vi "Edit_BSA_IP.vi"(3 "Show Panel":bool) -> (1 "Run LDA Diagnostic Out":bool)   [LabVIEW 2010]
uses:
  Globals/Meas_global.vi
  Globals/LDA_meas_global_1.vi
  Globals/LDA_meas_global_2.vi
panel:
  in  "Run LDA Diagnostic":bool
  in  "Bandwidth 0":u16(ring)=11 items=["96.777", "48.389", "24.194", "12.097", "6.049", "3.024", "1.512", "0.756", "0.378", "0.189", "0.095", "0.047"]
  in  "Centre frequency 1":u16(ring)=20 items=["5.378", "5.020", "4.661", "4.303", "3.944", "3.586", "3.227", "2.869", "2.510", "2.151", "1.793", "1.434", "1.076", "0.717", "0.359", "0.000", "-0.359", "-0.717", "-1.076", "-1.434", "-1.793", "-2.151", "-2.510", "-2.869", "-3.227", "-3.586", "-3.944", "-4.303", "-4.661", "-5.020", "-5.378", "-5.737", "-6.096"]
  out "Record Length":dbl[](array[numeric])
  out "Final read?":bool
  in  "OK":bool
  out "C Array":dbl[](array[numeric])
  out "Bandwidth Array Hz":dbl[](array[numeric])
  out "BSA IP Number":string
  out "Using 45 Degree Mirror?":bool
  out "Probe Configuration":string
  out "Focal Length (mm)":dbl
  out "Beam Separation (mm)":dbl
  in  "Bandwidth 1":u16(ring)=11 items=["91.793", "45.896", "22.948", "11.474", "5.737", "2.869", "1.434", "0.717", "0.359", "0.179", "0.090", "0.045"]
  in  "Centre frequency 0":u16(ring)=20 items=["5.671", "5.293", "4.914", "4.536", "4.158", "3.780", "3.402", "3.024", "2.646", "2.268", "1.890", "1.512", "1.134", "0.756", "0.378", "0.000", "-0.378", "-0.756", "-1.134", "-1.512", "-1.890", "-2.268", "-2.646", "-3.024", "-3.402", "-3.780", "-4.158", "-4.536", "-4.914", "-5.293", "-5.671", "-6.049", "-6.427"]
  in  "Setup Array":T1(array[cluster]) {"Bandwidth Hz" format="%.3g"; "Min Record length" items=["16", "32", "64", "128", "256"]; "Optics Conversion Factor" format="%.3g"; "High voltage" min=0 max=2040 step=8; "Signal gain (dB)" min=0 max=30 step=1; "Max Record length" items=["16", "32", "64", "128", "256"]; "Min Velocity" format="%.2g"; "Max Velocity" format="%.2g"; "Wavelength (nm)" format="%.1f"}
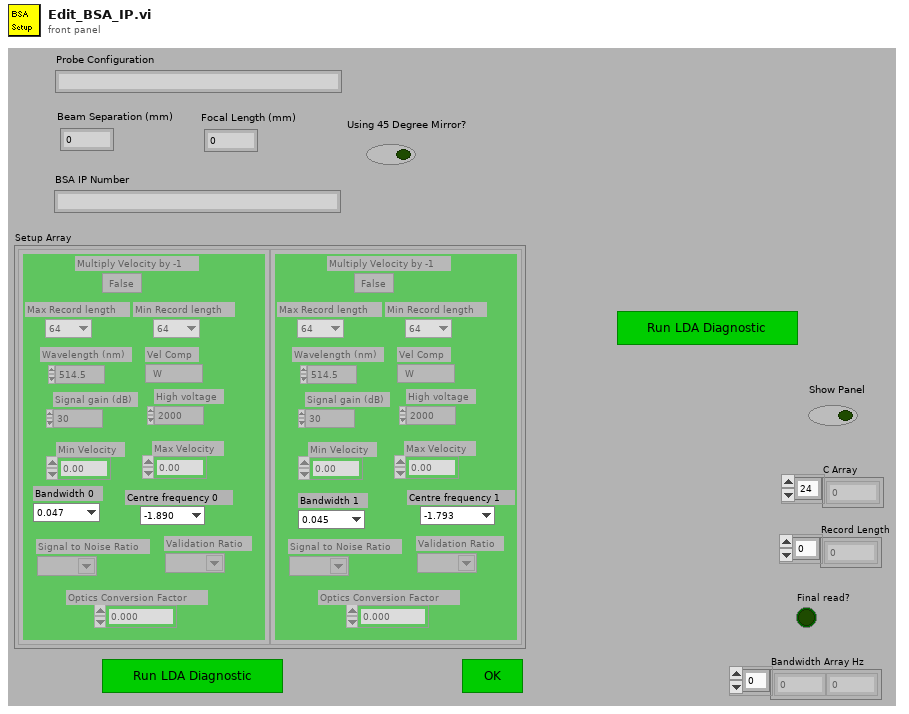
[diagram p1: front panel]
types:
  T1 = cluster{"Wavelength (nm)":dbl, "Vel Comp":string, "Max Velocity":dbl, "Min Velocity":dbl, "COLOUR":u32, "Max Record length":u16, "Signal gain (dB)":i16, "High voltage":i16, "Optics Conversion Factor":dbl, "Min Record length":u16, "Bandwidth Hz":dbl, "Multiply Velocity by -1":bool, "Signal to Noise Ratio":string, "Validation Ratio":string}[]
  T2 = cluster{"Wavelength (nm)":dbl, "Vel Comp":string, "Max Velocity":dbl, "Min Velocity":dbl, "COLOUR":u32, "Max Record length":u16, "Signal gain (dB)":i16, "High voltage":i16, "Optics Conversion Factor":dbl, "Min Record length":u16, "Bandwidth Hz":dbl, "Multiply Velocity by -1":bool, "Signal to Noise Ratio":string, "Validation Ratio":string}
  T3 = typedef "BSA_info_Cluster.ctl" = cluster{"GPIB Address":string, "No of Check Bytes":i32, "Extra Info":string, "COLOUR":u32, "Wavelength (nm)":dbl}
  T4 = typedef "BSA_Type.ctl" = enum16{"57N11", "BSA F60"}
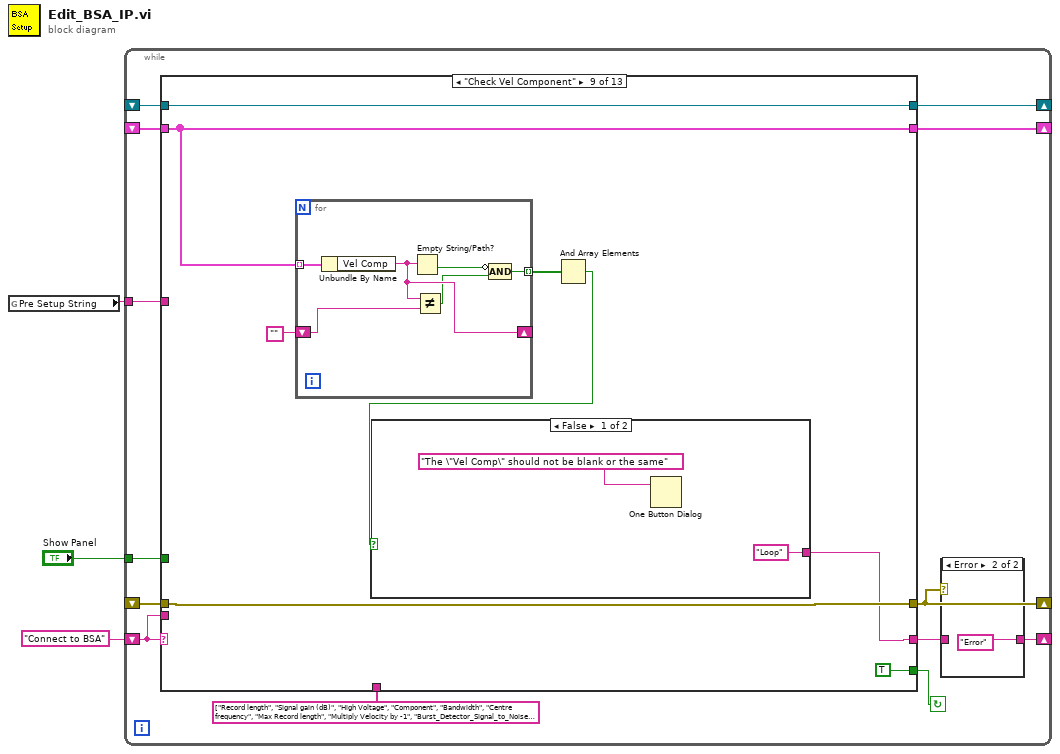
[diagram p0: block diagram]
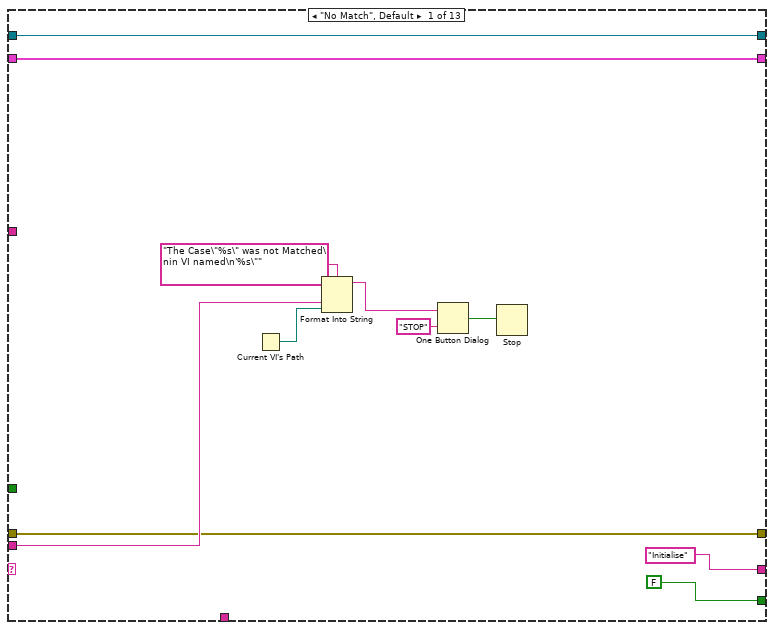
[diagram p3: hidden frame]
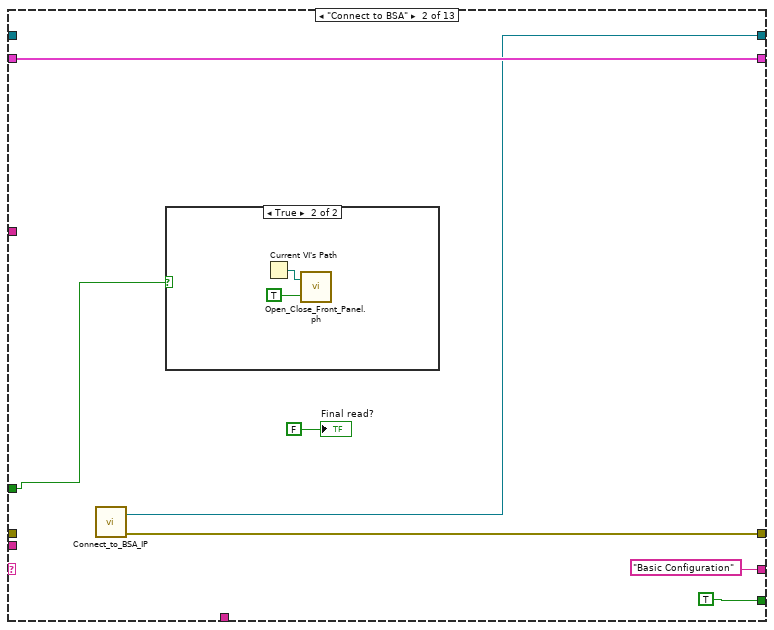
[diagram p4: hidden frame]
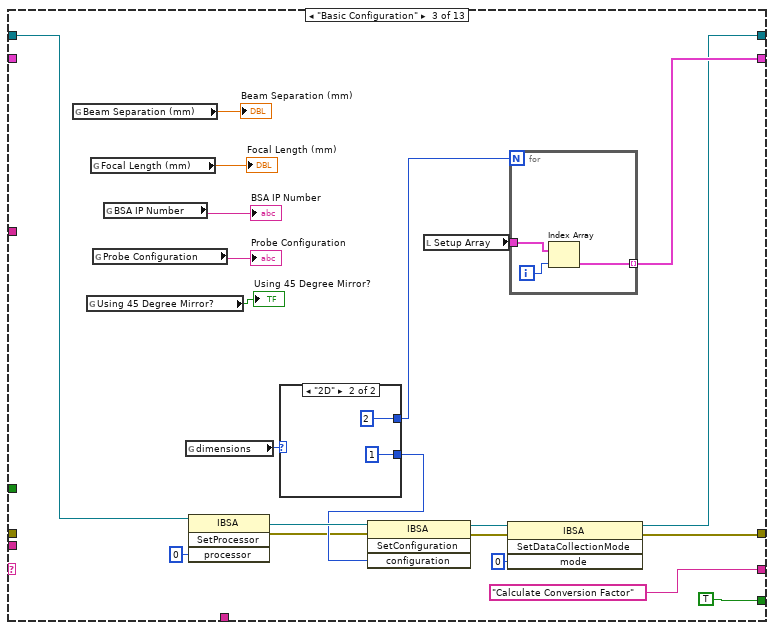
[diagram p6: hidden frame]
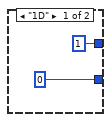
[diagram p7: hidden frame]
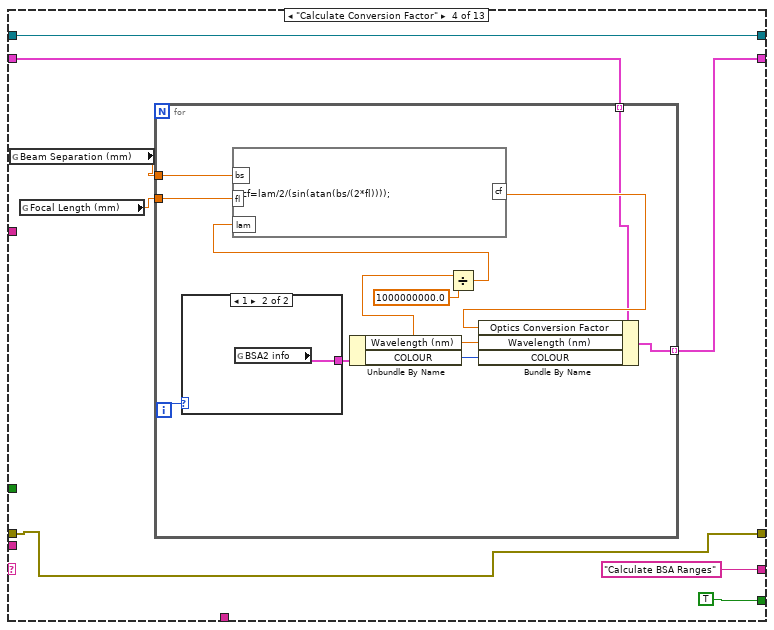
[diagram p8: hidden frame]
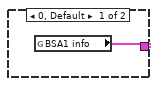
[diagram p9: hidden frame]
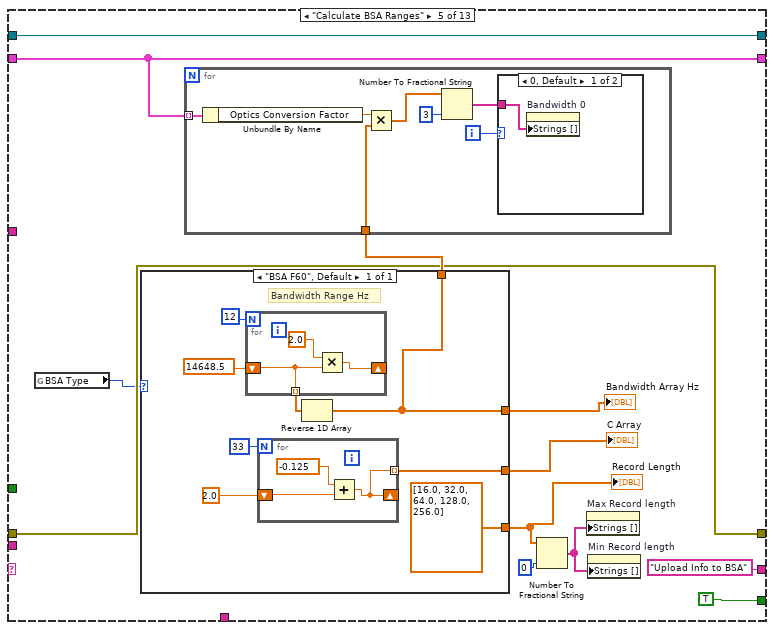
[diagram p10: hidden frame]
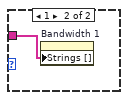
[diagram p11: hidden frame]
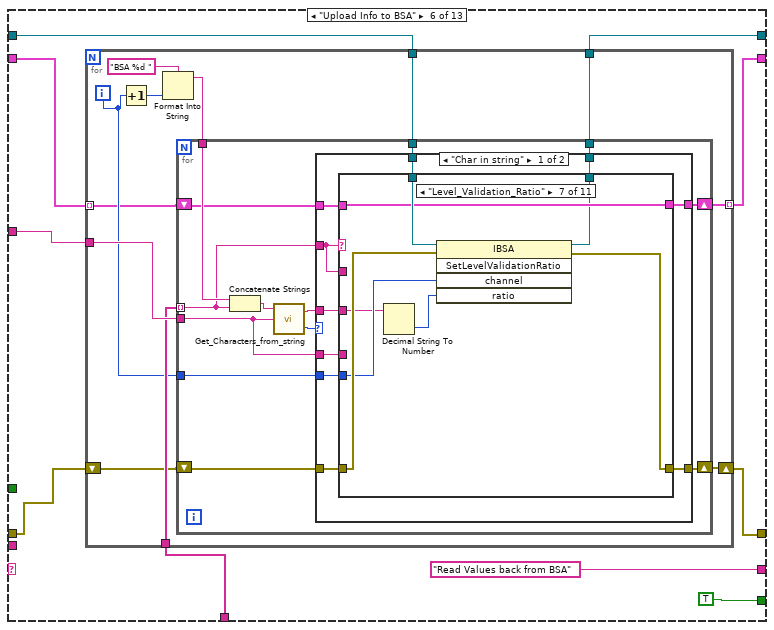
[diagram p12: hidden frame]
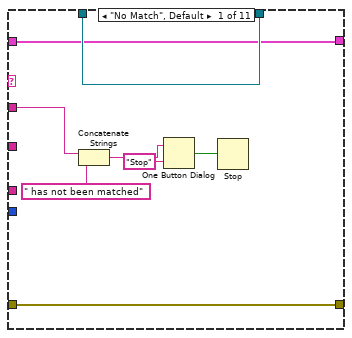
[diagram p13: hidden frame]
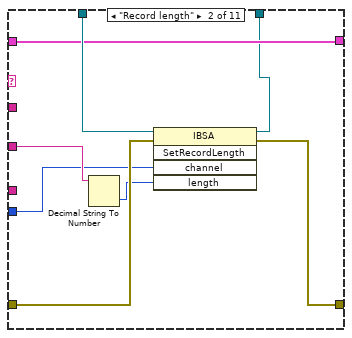
[diagram p14: hidden frame]
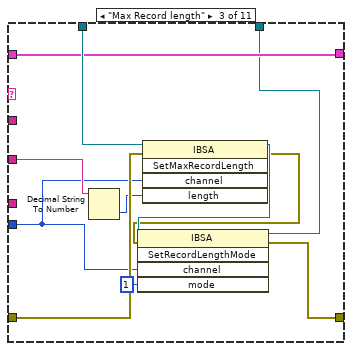
[diagram p15: hidden frame]
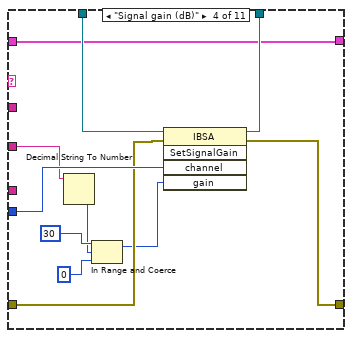
[diagram p16: hidden frame]
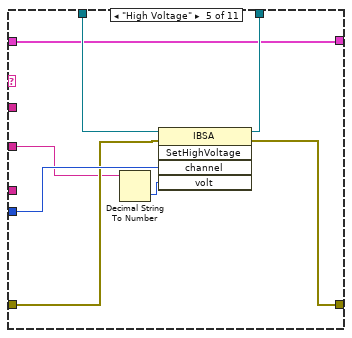
[diagram p17: hidden frame]
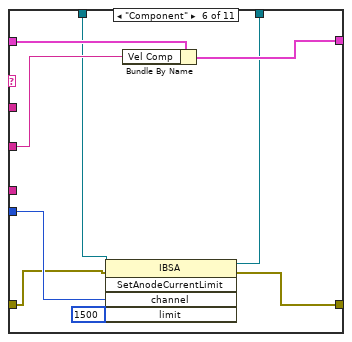
[diagram p18: hidden frame]
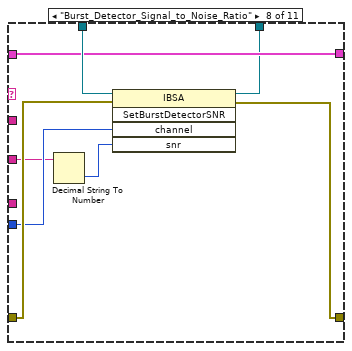
[diagram p19: hidden frame]
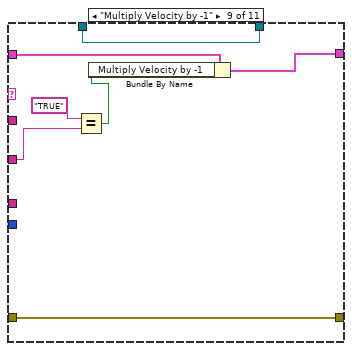
[diagram p20: hidden frame]
diagram:
  n1 = global read "Meas_global.vi" "Pre Setup String"() -> (w2:string)
  n2 = while {
    shift-left: "Connect to BSA" -> [w15]
    shift-right: [w13] -> _
    shift-right: [w11] -> _
    shift-left: _ -> [w9]
    shift-right: [w14] -> _
    shift-left: _ -> [w10]
    tunnel: w2 -> [w8]
    shift-right: [w7] -> _
    shift-left: _ -> [w6]
    tunnel: "Show Panel" -> [w4]
    stop <- w16 continue-if-true
    n3 = case shown="\"Check Vel Component\"" w15 {
      tunnel: [FALSE TRUE TRUE TRUE TRUE TRUE TRUE TRUE TRUE ("Show Panel") TRUE FALSE w609 FALSE] -> w16
      tunnel: ["Initialise" "Basic Configuration" "Calculate Conversion Factor" "Calculate BSA Ranges" "Upload Info to BSA" "Read Values back from BSA" w269 w406 w471 "Read Values back from BSA" "Second Case" "Close Panel" "End" ("f")] -> w12
      tunnel: w15 -> [w24 _ _ _ _ _ _ _ _ _ _ _ _]
      tunnel: [w20 w32 w40 w69 w95 w127 w276 w411 w473 w491 w604 w611 w672] -> w14
      tunnel: [w21 w33 w41 w70 w98 w129 w278 w416 w477 w493 w605 w613 w673] -> w11
      tunnel: w10 -> [w20 _ _ w69 w95 w128 w277 w411 w473 w492 w604 w611 w672]
      tunnel: w9 -> [w21 _ w53 w70 w98 w130 w279 w416 w477 w494 w605 w613 w673]
      tunnel: w8 -> [_ _ _ _ _ w131 w280 _ _ w495 _ _ _]
      tunnel: [w19 w34 w45 w71 w97 w125 w273 w412 w470 w489 w603 w612 w668] -> w7
      tunnel: w6 -> [w19 w34 _ w68 w97 w126 w275 _ w470 w490 w603 w612 w668]
      tunnel: string[] ["Record length", "Signal gain (dB)", "High Voltage", "Component", "Bandwidth", "Centre frequency", "Max Record length", "Multiply Velocity by -1", "Burst_Detector_Signal_to_Noise_Ratio", "Level_Validation_Ratio"] -> [_ _ _ _ _ w124 w274 _ _ w488 _ _ _]
      tunnel: w4 -> [_ w30 _ _ _ _ _ w403 _ _ _ w609 _]
      frame "No Match", Default {
        n4 = Current VI's Path() -> (path=w23:path)
        n5 = Format Into String(format string="The Case\"%s\" was not Matched\nin VI named\n'%s\"" ("Format String"), w24, w23) -> (resulting string=w27:string)  [unwired: 2 in, 1 out]
        n6 = One Button Dialog(message=w27, button name ("OK")="STOP") -> (true=w25:bool)
        n7 = Stop(stop? (T)=w25) -> ()
      }
      frame "Connect to BSA" {
        n8 = call "Connect_to_BSA_IP.vi"() -> ("error out"=w32:errorcluster, "BSA"=w33:refnum<k7>)  [unwired: 2 out]
        n9 = case shown="True" w30 {
          frame False {
          }
          frame True {
            n10 = Current VI's Path() -> (path=w37:path)
            n11 = call "Open_Close_Front_Panel.ph.vi"("Front Panel Window:Open"=TRUE, "VI path"=w37) -> ()  [unwired: 2 out]
          }
        }
        "Final read?" <- FALSE ("Boolean")
      }
      frame "Basic Configuration" {
        n12 = global read "LDA_meas_global_1.vi" "Beam Separation (mm)"() -> (→"Beam Separation (mm)":dbl)
        n13 = global read "LDA_meas_global_1.vi" "Using 45 Degree Mirror?"() -> (→"Using 45 Degree Mirror?":bool)
        n14 = global read "LDA_meas_global_1.vi" "Focal Length (mm)"() -> (→"Focal Length (mm)":dbl)
        n15 = global read "LDA_meas_global_1.vi" "Probe Configuration"() -> (→"Probe Configuration":string)
        n16 = global read "LDA_meas_global_1.vi" "BSA IP Number"() -> (→"BSA IP Number":string)
        n17 = global read "Meas_global.vi" "dimensions"() -> (w56:enum16{"1D", "2D"})
        n18 = invoke class="IBSA" method="SetProcessor"(reference=w53, "processor"=0) -> (reference out=w57:refnum<k7>, error out=w54:errorcluster)  [unwired: 2 in, 2 out]
        n19 = case shown="\"2D\"" w56 {
          tunnel: [0 ("config") 1 ("config")] -> w55
          tunnel: [1 2] -> w46
          frame "1D" {
          }
          frame "2D" {
          }
        }
        n20 = invoke class="IBSA" method="SetConfiguration"(reference=w57, error in=w54, "configuration"=w55) -> (reference out=w43:refnum<k7>, error out=w42:errorcluster)  [unwired: 1 in, 2 out]
        n21 = local read "Setup Array"() -> (w47:T1)
        n22 = invoke class="IBSA" method="SetDataCollectionMode"(reference=w43, error in=w42, "mode"=0) -> (reference out=w41:refnum<k7>, error out=w40:errorcluster)  [unwired: 1 in, 2 out]
        n23 = for {
          N: w46 -> [_]
          tunnel: w47 -> [w61]
          tunnel: [w60] -> w45 mode=indexing
          i -> [w62]
          n24 = Index Array(array=w61, index=w62) -> (element=w60:T2)
        }
      }
      frame "Calculate Conversion Factor" {
        n25 = global read "LDA_meas_global_1.vi" "Beam Separation (mm)"() -> (w72:dbl)
        n26 = global read "LDA_meas_global_1.vi" "Focal Length (mm)"() -> (w73:dbl)
        n27 = for {
          tunnel: w72 -> [w85]
          tunnel: w73 -> [w84]
          tunnel: [w76] -> w71 mode=indexing
          tunnel: w68 -> [w75] mode=indexing
          i -> [w82]
          n28 = case shown="1" w82 {
            tunnel: [w86 w87] -> w83
            frame 0, Default {
              n29 = global read "LDA_meas_global_1.vi" "BSA1 info"() -> (w86:T3)
            }
            frame 1 {
              n30 = global read "LDA_meas_global_2.vi" "BSA2 info"() -> (w87:T3)
            }
          }
          n31 = Unbundle By Name(w83) -> ("Wavelength (nm)"=w79:dbl, "COLOUR"=w81:u32)
          n32 = Divide(x=w79, y=1000000000.0) -> (x/y=w77:dbl)
          n33 = formula code="cf=lam/2/(sin(atan(bs/(2*fl))));"("bs"=w85, "fl"=w84, "lam"=w77) -> ("cf"=w80:dbl)
          n34 = Bundle By Name(cluster=w75, "Optics Conversion Factor"=w80, "Wavelength (nm)"=w79, "COLOUR"=w81) -> (w76:T2)
        }
      }
      frame "Calculate BSA Ranges" {
        n35 = global read "LDA_meas_global_1.vi" "BSA Type"() -> (w89:T4)
        n36 = case shown="\"BSA F60\", Default" w89 {
          tunnel: [w110] -> w96
          tunnel: [w111] -> w93
          tunnel: [w110] -> w92
          tunnel: [dbl[] [16.0, 32.0, 64.0, 128.0, 256.0] ("Max Record Length")] -> w90
          frame "BSA F60", Default {
            # "Bandwidth Range Hz"
            n37 = for {
              N: 12 -> [_]
              shift-right: [w122] -> _
              shift-left: 14648.5 -> [w120]
              tunnel: [w120] -> w114 mode=indexing
              n38 = Multiply(x=2.0, y=w120) -> (x*y=w122:dbl)
            }
            n39 = for {
              N: 33 -> [_]
              shift-right: [w117] -> _
              shift-left: 2.0 -> [w119]
              tunnel: [w117] -> w111 mode=indexing
              n40 = Add(x=-0.125, y=w119) -> (x+y=w117:dbl)
            }
            n41 = Reverse 1D Array(array=w114) -> (reversed array=w110:dbl[])
          }
        }
        "C Array" <- w93
        "Bandwidth Array Hz" <- w92
        "Record Length" <- w90
        n42 = for {
          tunnel: w97 -> [w106] mode=indexing
          tunnel: w96 -> [w104]
          i -> [w105]
          n43 = Unbundle By Name(w106) -> ("Optics Conversion Factor"=w100:dbl)
          n44 = Multiply(x=w100, y=w104) -> (x*y=w103:dbl[])
          n45 = Number To Fractional String(number=w103, precision (6)=i16 3) -> (F-format string=w101:string[])  [unwired: 2 out]
          n46 = case shown="0, Default" w105 {
            tunnel: w101 -> [w107 w108]
            frame 0, Default {
              n47 = property on="Bandwidth 0" class="Ring (strict)"("Strings []"=w107) -> ()  [unwired: 2 in, 2 out]
            }
            frame 1 {
              n48 = property on="Bandwidth 1" class="Ring (strict)"("Strings []"=w108) -> ()  [unwired: 2 in, 2 out]
            }
          }
        }
        n49 = Number To Fractional String(number=w90, precision (6)=i16 0) -> (F-format string=w88:string[])  [unwired: 2 out]
        n50 = property on="Max Record length" class="Ring (strict)"("Strings []"=w88) -> ()  [unwired: 2 in, 2 out]
        n51 = property on="Min Record length" class="Ring (strict)"("Strings []"=w88) -> ()  [unwired: 2 in, 2 out]
      }
      frame "Upload Info to BSA" {
        n52 = for {
          tunnel: w131 -> [w144]
          tunnel: w130 -> [w143]
          tunnel: [w142] -> w129
          shift-right: [w139] -> w127
          shift-left: w128 -> [w140]
          tunnel: w124 -> [w141]
          tunnel: w126 -> [w134] mode=indexing
          tunnel: [w133] -> w125 mode=indexing
          i -> [w138]
          n53 = Increment(x=w138) -> (x+1=w137:i32)
          n54 = Format Into String(format string="BSA %d ", w137) -> (resulting string=w135:string)  [unwired: 2 in, 1 out]
          n55 = for {
            tunnel: w135 -> [w157]
            tunnel: w138 -> [w156]
            tunnel: w144 -> [w149]
            tunnel: w143 -> [w155]
            tunnel: [w154] -> w142
            tunnel: w141 -> [w153] mode=indexing
            shift-right: [w151] -> w139
            shift-left: w140 -> [w152]
            shift-right: [w145] -> w133
            shift-left: w134 -> [w146]
            n56 = Concatenate Strings(w157, w153) -> (w150:string)
            n57 = call "Get_Characters_from_string.vi"("Input string"=w149, "Variable name"=w150) -> ("Status"=w148:enum16{"Char in string", "Char not in string"}, "Value"=w147:string)  [unwired: 1 in]
            n58 = case shown="\"Char in string\"" w148 {
              tunnel: w156 -> [w167 _]
              tunnel: w147 -> [w166 _]
              tunnel: w153 -> [w161 _]
              tunnel: w155 -> [w165 w268]
              tunnel: [w164 w268] -> w154
              tunnel: [w163 w267] -> w151
              tunnel: w152 -> [w162 w267]
              tunnel: w146 -> [w160 w266]
              tunnel: w149 -> [w159 _]
              tunnel: [w158 w266] -> w145
              frame "Char in string" {
                n59 = case shown="\"Level_Validation_Ratio\"" w161 {
                  tunnel: w167 -> [_ w178 w188 w205 w213 w219 w228 w236 _ w255 w265]
                  tunnel: w166 -> [_ w181 w192 w200 w207 w221 w226 w234 w243 w250 w260]
                  tunnel: w165 -> [w175 w183 w194 w204 w212 w215 w230 w238 w239 w254 w264]
                  tunnel: [w175 w177 w184 w203 w211 w216 w223 w231 w239 w253 w263] -> w164
                  tunnel: [w174 w176 w185 w202 w210 w217 w224 w232 w240 w252 w262] -> w163
                  tunnel: w162 -> [w174 w182 w193 w201 w209 w214 w229 w237 w240 w251 w261]
                  tunnel: w161 -> [w173 _ _ _ _ _ _ _ _ _ _]
                  tunnel: w160 -> [w168 w180 w191 w199 w206 w222 w227 w235 w245 w248 w258]
                  tunnel: w159 -> [_ _ _ _ _ _ _ _ _ _ _]
                  tunnel: [w168 w180 w191 w199 w206 w220 w227 w235 w244 w248 w258] -> w158
                  frame "No Match", Default {
                    n60 = Concatenate Strings(w173, " has not been matched" ("string")) -> (w171:string)
                    n61 = One Button Dialog(message=w171, button name ("OK")="Stop") -> (true=w169:bool)
                    n62 = Stop(stop? (T)=w169) -> ()
                  }
                  frame "Record length" {
                    n63 = Decimal String To Number(string=w181) -> (number=w179:i32)  [unwired: 3 out]
                    n64 = invoke class="IBSA" method="SetRecordLength"(reference=w183, error in=w182, "channel"=w178, "length"=w179) -> (reference out=w177:refnum<k7>, error out=w176:errorcluster)  [unwired: 1 in, 3 out]
                  }
                  frame "Max Record length" {
                    n65 = Decimal String To Number(string=w192) -> (number=w190:i32)  [unwired: 3 out]
                    n66 = invoke class="IBSA" method="SetMaxRecordLength"(reference=w194, error in=w193, "channel"=w188, "length"=w190) -> (reference out=w187:refnum<k7>, error out=w186:errorcluster)  [unwired: 1 in, 3 out]
                    n67 = invoke class="IBSA" method="SetRecordLengthMode"(reference=w187, error in=w186, "channel"=w188, "mode"=1) -> (reference out=w184:refnum<k7>, error out=w185:errorcluster)  [unwired: 1 in, 3 out]
                  }
                  frame "Signal gain (dB)" {
                    n68 = Decimal String To Number(string=w200) -> (number=w195:i32)  [unwired: 3 out]
                    n69 = In Range and Coerce(upper limit=30, x=w195, lower limit=0) -> (coerced(x)=w196:i32)  [unwired: 1 out]
                    n70 = invoke class="IBSA" method="SetSignalGain"(reference=w204, error in=w201, "channel"=w205, "gain"=w196) -> (reference out=w203:refnum<k7>, error out=w202:errorcluster)  [unwired: 1 in, 3 out]
                  }
                  frame "High Voltage" {
                    n71 = Decimal String To Number(string=w207) -> (number=w208:i32)  [unwired: 3 out]
                    n72 = invoke class="IBSA" method="SetHighVoltage"(reference=w212, error in=w209, "channel"=w213, "volt"=w208) -> (reference out=w211:refnum<k7>, error out=w210:errorcluster)  [unwired: 1 in, 3 out]
                  }
                  frame "Component" {
                    n73 = invoke class="IBSA" method="SetAnodeCurrentLimit"(reference=w215, error in=w214, "channel"=w219, "limit"=1500) -> (reference out=w216:refnum<k7>, error out=w217:errorcluster)  [unwired: 1 in, 3 out]
                    n74 = Bundle By Name(cluster=w222, "Vel Comp"=w221) -> (w220:T2)
                  }
                  frame "Level_Validation_Ratio" {
                    n75 = Decimal String To Number(string=w226) -> (number=w225:i32)  [unwired: 3 out]
                    n76 = invoke class="IBSA" method="SetLevelValidationRatio"(reference=w230, error in=w229, "channel"=w228, "ratio"=w225) -> (reference out=w223:refnum<k7>, error out=w224:errorcluster)  [unwired: 1 in, 3 out]
                  }
                  frame "Burst_Detector_Signal_to_Noise_Ratio" {
                    n77 = Decimal String To Number(string=w234) -> (number=w233:i32)  [unwired: 3 out]
                    n78 = invoke class="IBSA" method="SetBurstDetectorSNR"(reference=w238, error in=w237, "channel"=w236, "snr"=w233) -> (reference out=w231:refnum<k7>, error out=w232:errorcluster)  [unwired: 1 in, 3 out]
                  }
                  frame "Multiply Velocity by -1" {
                    n79 = Equal?(x="TRUE", y=w243) -> (x = y?=w241:bool)
                    n80 = Bundle By Name(cluster=w245, "Multiply Velocity by -1"=w241) -> (w244:T2)
                  }
                  frame "Bandwidth" {
                    n81 = Fract/Exp String To Number(string=w250) -> (number=w249:dbl)  [unwired: 4 out]
                    n82 = Unbundle By Name(w248) -> ("Optics Conversion Factor"=w247:dbl)
                    n83 = Divide(x=w249, y=w247) -> (x/y=w246:dbl)
                    n84 = invoke class="IBSA" method="SetBandwidth"(reference=w254, error in=w251, "channel"=w255, "bandwidth"=w246) -> (reference out=w253:refnum<k7>, error out=w252:errorcluster)  [unwired: 1 in, 3 out]
                  }
                  frame "Centre frequency" {
                    n85 = Fract/Exp String To Number(string=w260) -> (number=w259:dbl)  [unwired: 4 out]
                    n86 = Unbundle By Name(w258) -> ("Optics Conversion Factor"=w257:dbl)
                    n87 = Divide(x=w259, y=w257) -> (x/y=w256:dbl)
                    n88 = invoke class="IBSA" method="SetCenterFreq"(reference=w264, error in=w261, "channel"=w265, "freq"=w256) -> (reference out=w263:refnum<k7>, error out=w262:errorcluster)  [unwired: 1 in, 3 out]
                  }
                }
              }
              frame "Char not in string" {
              }
            }
          }
        }
      }
      frame "Read Values back from BSA" {
        n89 = for {
          tunnel: w280 -> [w290]
          tunnel: w279 -> [w289]
          tunnel: [w288] -> w278
          shift-right: [w285] -> w276
          shift-left: w277 -> [w286]
          tunnel: w274 -> [w287]
          tunnel: w275 -> [w284] mode=indexing
          tunnel: [w283] -> w273 mode=indexing
          i -> [w282]
          n90 = for {
            tunnel: w282 -> [w299]
            tunnel: w290 -> [w293]
            tunnel: w289 -> [w298]
            tunnel: [w297] -> w288
            tunnel: w287 -> [w296] mode=indexing
            shift-right: [w294] -> w285
            shift-left: w286 -> [w295]
            shift-right: [w291] -> w283
            shift-left: w284 -> [w292]
            n91 = case shown="\"Level_Validation_Ratio\"" w296 {
              tunnel: w299 -> [_ w319 w331 w339 w348 w357 w365 _ _ w379 w394]
              tunnel: w298 -> [w307 w318 w330 w338 w347 w356 w364 w367 w370 w383 w398]
              tunnel: [w307 w317 w329 w337 w346 w355 w363 w367 w370 w382 w397] -> w297
              tunnel: [w306 w316 w328 w336 w345 w354 w362 w368 w371 w381 w396] -> w294
              tunnel: w295 -> [w306 w315 w327 w335 w344 w353 w361 w368 w371 w380 w395]
              tunnel: w296 -> [w305 _ _ _ _ _ _ _ _ _ _]
              tunnel: w292 -> [w300 w314 w326 w333 w343 w352 w360 w366 w369 w374 w390]
              tunnel: w293 -> [_ _ _ _ _ _ _ _ _ _ _]
              tunnel: [w300 w313 w325 w332 w342 w351 w359 w366 w369 w372 w390] -> w291
              frame "No Match", Default {
                n92 = Concatenate Strings(w305, " has not been matched" ("string")) -> (w303:string)
                n93 = One Button Dialog(message=w303, button name ("OK")="Stop") -> (true=w301:bool)
                n94 = Stop(stop? (T)=w301) -> ()
              }
              frame "Record length" {
                n95 = local read "Record Length"() -> (w310:dbl[])
                n96 = invoke class="IBSA" method="GetRecordLength"(reference=w318, error in=w315, "channel"=w319) -> (reference out=w317:refnum<k7>, error out=w316:errorcluster, "GetRecordLength"=w309:i32)  [unwired: 1 in, 1 out]
                n97 = Subtract(x=w310, y=w309) -> (x-y=w312:dbl[])
                n98 = Absolute Value(x=w312) -> (abs(x)=w311:dbl[])
                n99 = Array Max & Min(array=w311) -> (min index (indices)=w308:i32)  [unwired: 3 out]
                n100 = Bundle By Name(cluster=w314, "Min Record length"=w308) -> (w313:T2)
              }
              frame "Max Record length" {
                n101 = local read "Record Length"() -> (w322:dbl[])
                n102 = invoke class="IBSA" method="GetMaxRecordLength"(reference=w330, error in=w327, "channel"=w331) -> (reference out=w329:refnum<k7>, error out=w328:errorcluster, "GetMaxRecordLength"=w321:i32)  [unwired: 1 in, 1 out]
                n103 = Subtract(x=w322, y=w321) -> (x-y=w324:dbl[])
                n104 = Absolute Value(x=w324) -> (abs(x)=w323:dbl[])
                n105 = Array Max & Min(array=w323) -> (min index (indices)=w320:i32)  [unwired: 3 out]
                n106 = Bundle By Name(cluster=w326, "Max Record length"=w320) -> (w325:T2)
              }
              frame "Signal gain (dB)" {
                n107 = invoke class="IBSA" method="GetSignalGain"(reference=w338, error in=w335, "channel"=w339) -> (reference out=w337:refnum<k7>, error out=w336:errorcluster, "GetSignalGain"=w334:i32)  [unwired: 1 in, 1 out]
                n108 = Bundle By Name(cluster=w333, "Signal gain (dB)"=w334) -> (w332:T2)
              }
              frame "Burst_Detector_Signal_to_Noise_Ratio" {
                n109 = invoke class="IBSA" method="GetBurstDetectorSNR"(reference=w347, error in=w344, "channel"=w348) -> (reference out=w346:refnum<k7>, error out=w345:errorcluster, "GetBurstDetectorSNR"=w340:i32)  [unwired: 1 in, 1 out]
                n110 = Number To Decimal String(number=w340) -> (decimal integer string=w341:string)  [unwired: 1 out]
                n111 = Bundle By Name(cluster=w343, "Signal to Noise Ratio"=w341) -> (w342:T2)
              }
              frame "Level_Validation_Ratio" {
                n112 = invoke class="IBSA" method="GetLevelValidationRatio"(reference=w356, error in=w353, "channel"=w357) -> (reference out=w355:refnum<k7>, error out=w354:errorcluster, "GetLevelValidationRatio"=w349:i32)  [unwired: 1 in, 1 out]
                n113 = Number To Decimal String(number=w349) -> (decimal integer string=w350:string)  [unwired: 1 out]
                n114 = Bundle By Name(cluster=w352, "Validation Ratio"=w350) -> (w351:T2)
              }
              frame "High Voltage" {
                n115 = invoke class="IBSA" method="GetHighVoltage"(reference=w364, error in=w361, "channel"=w365) -> (reference out=w363:refnum<k7>, error out=w362:errorcluster, "GetHighVoltage"=w358:i32)  [unwired: 1 in, 1 out]
                n116 = Bundle By Name(cluster=w360, "High voltage"=w358) -> (w359:T2)
              }
              frame "Component" {
              }
              frame "Multiply Velocity by -1" {
              }
              frame "Bandwidth" {
                n117 = local read "Bandwidth Array Hz"() -> (w376:dbl[])
                n118 = invoke class="IBSA" method="GetBandwidth"(reference=w383, error in=w380, "channel"=w379) -> (reference out=w382:refnum<k7>, error out=w381:errorcluster, "GetBandwidth"=w373:sgl)  [unwired: 1 in, 1 out]
                n119 = Bundle By Name(cluster=w374, "Bandwidth Hz"=w373) -> (w372:T2)
                n120 = Subtract(x=w376, y=w373) -> (x-y=w378:dbl[])
                n121 = Absolute Value(x=w378) -> (abs(x)=w377:dbl[])
                n122 = Array Max & Min(array=w377) -> (min index (indices)=w375:i32)  [unwired: 3 out]
                n123 = case shown="1" w379 {
                  tunnel: w375 -> [w384 w385]
                  frame 0, Default {
                    n124 = local write "Bandwidth 0"(w384) -> ()
                  }
                  frame 1 {
                    n125 = local write "Bandwidth 1"(w385) -> ()
                  }
                }
              }
              frame "Centre frequency" {
                n126 = local read "C Array"() -> (w389:dbl[])
                n127 = Unbundle By Name(w390) -> ("Bandwidth Hz"=w387:dbl)
                n128 = invoke class="IBSA" method="GetCenterFreq"(reference=w398, error in=w395, "channel"=w394) -> (reference out=w397:refnum<k7>, error out=w396:errorcluster, "GetCenterFreq"=w388:sgl)  [unwired: 1 in, 1 out]
                n129 = Divide(x=w388, y=w387) -> (x/y=w386:dbl)
                n130 = Subtract(x=w389, y=w386) -> (x-y=w393:dbl[])
                n131 = Absolute Value(x=w393) -> (abs(x)=w392:dbl[])
                n132 = Array Max & Min(array=w392) -> (min index (indices)=w391:i32)  [unwired: 3 out]
                n133 = case shown="1" w394 {
                  tunnel: w391 -> [w399 w400]
                  frame 0, Default {
                    n134 = local write "Centre frequency 0"(w399) -> ()
                  }
                  frame 1 {
                    n135 = local write "Centre frequency 1"(w400) -> ()
                  }
                }
              }
            }
          }
        }
        n136 = local read "Final read?"() -> (w272:bool)
        n137 = local write "Setup Array"(w273) -> ()
        n138 = Select(t="Update Globals", s=w272, f="Loop") -> (s? t:f=w269:string)
      }
      frame "Loop" {
        n139 = local read "Bandwidth Array Hz"() -> (w415:dbl[])
        n140 = local read "C Array"() -> (w414:dbl[])
        n141 = Wait Until Next ms Multiple(millisecond multiple=u32 300) -> ()  [unwired: 1 out]
        n142 = for {
          tunnel: w415 -> [w445]
          tunnel: w414 -> [w427]
          tunnel: [w442] -> w412 mode=indexing
          tunnel: "Setup Array" -> [w432] mode=indexing
          i -> [w441]
          n143 = Unbundle By Name(w432) -> ("Optics Conversion Factor"=w440:dbl, "Max Record length"=w433:u16, "Min Record length"=w435:u16, "Multiply Velocity by -1"=w426:bool)
          n144 = case shown="1" w441 {
            tunnel: ["Bandwidth 0" "Bandwidth 1"] -> w446
            tunnel: ["Centre frequency 0" "Centre frequency 1"] -> w444
            frame 0, Default {
            }
            frame 1 {
            }
          }
          n145 = Greater Or Equal?(x=w433, y=w435) -> (x >= y?=w434:bool)
          n146 = case shown="False" w434 {
            tunnel: w432 -> [w458 w459]
            tunnel: w433 -> [w457 _]
            tunnel: [w456 w459] -> w431
            frame False {
              n147 = Bundle By Name(cluster=w458, "Min Record length"=w457) -> (w456:T2)
            }
            frame True {
            }
          }
          n148 = Index Array(array=w445, index=w446) -> (element=w439:dbl)
          n149 = Multiply(x=w440, y=w439) -> (x*y=w437:dbl)
          n150 = Multiply(x=w427, y=w437) -> (x*y=w423:dbl[])
          n151 = Index Array(array=w423, index=w444) -> (element=w428:dbl)
          n152 = Divide(x=w437, y=2.0) -> (x/y=w429:dbl)
          n153 = Negate(x=w429) -> (-x=w430:dbl)
          n154 = Add(x=w430, y=w428) -> (x+y=w424:dbl)
          n155 = Add(x=w429, y=w428) -> (x+y=w425:dbl)
          n156 = case shown="False" w426 {
            tunnel: [w447 w453] -> w418
            tunnel: w425 -> [w447 w455]
            tunnel: [w449 w452] -> w419
            tunnel: w424 -> [w449 w454]
            tunnel: w423 -> [w448 w451]
            tunnel: [w448 w450] -> w422
            frame False {
            }
            frame True {
              n157 = Negate(x=w454) -> (-x=w452:dbl)
              n158 = Negate(x=w455) -> (-x=w453:dbl)
              n159 = Negate(x=w451) -> (-x=w450:dbl[])
            }
          }
          n160 = Max & Min(x=w419, y=w418) -> (max(x,y)=w420:dbl, min(x,y)=w421:dbl)
          n161 = Bundle By Name(cluster=w431, "Max Velocity"=w420, "Min Velocity"=w421) -> (w442:T2)
          n162 = Number To Fractional String(number=w422, precision (6)=i16 3) -> (F-format string=w436:string[])  [unwired: 2 out]
          n163 = case shown="1" w441 {
            tunnel: w437 -> [w462 w465]
            tunnel: w428 -> [w461 w464]
            tunnel: w436 -> [w460 w463]
            frame 0, Default {
              n164 = global write "LDA_meas_global_1.vi" "Centre Freq BSA1"(w461) -> ()
              n165 = global write "LDA_meas_global_1.vi" "Bandwidth BSA1"(w462) -> ()
              n166 = property on="Centre frequency 0" class="Ring (strict)"("Strings []"=w460) -> ()  [unwired: 2 in, 2 out]
            }
            frame 1 {
              n167 = global write "LDA_meas_global_2.vi" "Centre Freq BSA2"(w464) -> ()
              n168 = global write "LDA_meas_global_2.vi" "Bandwidth BSA2"(w465) -> ()
              n169 = property on="Centre frequency 1" class="Ring (strict)"("Strings []"=w463) -> ()  [unwired: 2 in, 2 out]
            }
          }
        }
        n170 = Not Equal?(x=w412, y="Setup Array") -> (x != y?=w413:bool)
        n171 = case shown="True" w413 {
          tunnel: w412 -> [_ w417]
          frame False {
          }
          frame True {
            n172 = local write "Setup Array"(w417) -> ()
          }
        }
        n173 = Compound Arithmetic op=AND(invert "Run LDA Diagnostic", invert "OK", w403) -> (w407:bool)
        n174 = Select(t="Loop", s=w407, f="Check Vel Component") -> (s? t:f=w406:string)
        "Run LDA Diagnostic Out" <- "Run LDA Diagnostic"
      }
      frame "Check Vel Component" {
        n175 = for {
          tunnel: w470 -> [w486] mode=indexing
          shift-right: [w484] -> _
          shift-left: "" -> [w485]
          tunnel: [w481] -> w475 mode=indexing
          n176 = Unbundle By Name(w486) -> ("Vel Comp"=w484:string)
          n177 = Empty String/Path?(string/path=w484) -> (empty?=w483:bool)
          n178 = Not Equal?(x=w484, y=w485) -> (x != y?=w482:bool)
          n179 = Compound Arithmetic op=AND(invert w483, w482) -> (w481:bool)
        }
        n180 = And Array Elements(Boolean array=w475) -> (logical AND=w474:bool)
        n181 = case shown="False" w474 {
          tunnel: ["Loop" "Write Setup to BSA" ("f")] -> w471
          frame False {
            n182 = One Button Dialog(message="The \"Vel Comp\" should not be blank or the same") -> ()  [unwired: 1 in, 1 out]
          }
          frame True {
          }
        }
      }
      frame "Write Setup to BSA" {
        n183 = for {
          tunnel: w495 -> [w506]
          tunnel: w494 -> [w505]
          tunnel: [w504] -> w493
          shift-right: [w501] -> w491
          shift-left: w492 -> [w502]
          tunnel: w488 -> [w503]
          tunnel: w490 -> [w499] mode=indexing
          tunnel: [w498] -> w489 mode=indexing
          i -> [w500]
          n184 = for {
            tunnel: w500 -> [w515]
            tunnel: w506 -> [w509]
            tunnel: w505 -> [w514]
            tunnel: [w513] -> w504
            tunnel: w503 -> [w512] mode=indexing
            shift-right: [w510] -> w501
            shift-left: w502 -> [w511]
            shift-right: [w507] -> w498
            shift-left: w499 -> [w508]
            n185 = case shown="\"Burst_Detector_Signal_to_Noise_Ratio\"" w512 {
              tunnel: w515 -> [_ w532 w541 w548 w555 w563 w571 _ _ w583 w595]
              tunnel: w514 -> [w523 w531 w540 w547 w554 w562 w570 w573 w576 w587 w600]
              tunnel: [w523 w530 w539 w546 w553 w561 w569 w573 w576 w586 w599] -> w513
              tunnel: [w522 w529 w538 w545 w552 w560 w568 w574 w577 w585 w598] -> w510
              tunnel: w511 -> [w522 w528 w537 w544 w551 w559 w567 w574 w577 w584 w597]
              tunnel: w512 -> [w521 _ _ _ _ _ _ _ _ _ _]
              tunnel: w508 -> [w516 w527 w536 w543 w550 w558 w566 w572 w575 w580 w596]
              tunnel: w509 -> [_ _ _ _ _ _ _ _ _ _ _]
              tunnel: [w516 w527 w536 w543 w550 w558 w566 w572 w575 w579 w596] -> w507
              frame "No Match", Default {
                n186 = Concatenate Strings(w521, " has not been matched" ("string")) -> (w519:string)
                n187 = One Button Dialog(message=w519, button name ("OK")="Stop") -> (true=w517:bool)
                n188 = Stop(stop? (T)=w517) -> ()
              }
              frame "Record length" {
                n189 = Unbundle By Name(w527) -> ("Min Record length"=w525:u16)
                n190 = local read "Record Length"() -> (w526:dbl[])
                n191 = Index Array(array=w526, index=w525) -> (element=w524:dbl)
                n192 = invoke class="IBSA" method="SetRecordLength"(reference=w531, error in=w528, "channel"=w532, "length"=w524) -> (reference out=w530:refnum<k7>, error out=w529:errorcluster)  [unwired: 1 in, 3 out]
              }
              frame "Max Record length" {
                n193 = Unbundle By Name(w536) -> ("Max Record length"=w534:u16)
                n194 = local read "Record Length"() -> (w535:dbl[])
                n195 = Index Array(array=w535, index=w534) -> (element=w533:dbl)
                n196 = invoke class="IBSA" method="SetMaxRecordLength"(reference=w540, error in=w537, "channel"=w541, "length"=w533) -> (reference out=w539:refnum<k7>, error out=w538:errorcluster)  [unwired: 1 in, 3 out]
              }
              frame "Signal gain (dB)" {
                n197 = Unbundle By Name(w543) -> ("Signal gain (dB)"=w542:i16)
                n198 = invoke class="IBSA" method="SetSignalGain"(reference=w547, error in=w544, "channel"=w548, "gain"=w542) -> (reference out=w546:refnum<k7>, error out=w545:errorcluster)  [unwired: 1 in, 3 out]
              }
              frame "High Voltage" {
                n199 = Unbundle By Name(w550) -> ("High voltage"=w549:i16)
                n200 = invoke class="IBSA" method="SetHighVoltage"(reference=w554, error in=w551, "channel"=w555, "volt"=w549) -> (reference out=w553:refnum<k7>, error out=w552:errorcluster)  [unwired: 1 in, 3 out]
              }
              frame "Level_Validation_Ratio" {
                n201 = Unbundle By Name(w558) -> ("Validation Ratio"=w557:string)
                n202 = Decimal String To Number(string=w557) -> (number=w556:i32)  [unwired: 3 out]
                n203 = invoke class="IBSA" method="SetLevelValidationRatio"(reference=w562, error in=w559, "channel"=w563, "ratio"=w556) -> (reference out=w561:refnum<k7>, error out=w560:errorcluster)  [unwired: 1 in, 3 out]
              }
              frame "Burst_Detector_Signal_to_Noise_Ratio" {
                n204 = Unbundle By Name(w566) -> ("Signal to Noise Ratio"=w565:string)
                n205 = Decimal String To Number(string=w565) -> (number=w564:i32)  [unwired: 3 out]
                n206 = invoke class="IBSA" method="SetBurstDetectorSNR"(reference=w570, error in=w567, "channel"=w571, "snr"=w564) -> (reference out=w569:refnum<k7>, error out=w568:errorcluster)  [unwired: 1 in, 3 out]
              }
              frame "Component" {
              }
              frame "Multiply Velocity by -1" {
              }
              frame "Bandwidth" {
                n207 = case shown="1" w583 {
                  tunnel: [w588 w589] -> w582
                  frame 0, Default {
                    n208 = local read "Bandwidth 0"() -> (w588:u16)
                  }
                  frame 1 {
                    n209 = local read "Bandwidth 1"() -> (w589:u16)
                  }
                }
                n210 = local read "Bandwidth Array Hz"() -> (w581:dbl[])
                n211 = Index Array(array=w581, index=w582) -> (element=w578:dbl)
                n212 = Bundle By Name(cluster=w580, "Bandwidth Hz"=w578) -> (w579:T2)
                n213 = invoke class="IBSA" method="SetBandwidth"(reference=w587, error in=w584, "channel"=w583, "bandwidth"=w578) -> (reference out=w586:refnum<k7>, error out=w585:errorcluster)  [unwired: 1 in, 3 out]
              }
              frame "Centre frequency" {
                n214 = case shown="1" w595 {
                  tunnel: [w601 w602] -> w594
                  frame 0, Default {
                    n215 = local read "Centre frequency 0"() -> (w601:u16)
                  }
                  frame 1 {
                    n216 = local read "Centre frequency 1"() -> (w602:u16)
                  }
                }
                n217 = Unbundle By Name(w596) -> ("Bandwidth Hz"=w591:dbl)
                n218 = local read "C Array"() -> (w593:dbl[])
                n219 = Index Array(array=w593, index=w594) -> (element=w592:dbl)
                n220 = Multiply(x=w591, y=w592) -> (x*y=w590:dbl)
                n221 = invoke class="IBSA" method="SetCenterFreq"(reference=w600, error in=w597, "channel"=w595, "freq"=w590) -> (reference out=w599:refnum<k7>, error out=w598:errorcluster)  [unwired: 1 in, 3 out]
              }
            }
          }
        }
        n222 = local write "Final read?"(TRUE ("Boolean")) -> ()
      }
      frame "Error" {
        n223 = call "EnFlo_Error_Handler.vi"("error in (no error)"=w604, "Dialog Box (T)"=TRUE) -> ()  [unwired: 1 in, 3 out]
      }
      frame "Update Globals" {
        n224 = for {
          tunnel: w612 -> [w615] mode=indexing
          i -> [w614]
          n225 = stacked-sequence {
            seq-local: [w616 _] -> [_ w632]
            tunnel: w615 -> [w631 w646]
            tunnel: w614 -> [w626 w633]
            frame #0 {
              n226 = Increment(x=w626) -> (x+1=w629:i32)
              n227 = Unbundle By Name(w631) -> ("Signal to Noise Ratio"=w623:string, "Validation Ratio"=w620:string)
              n228 = Number To Decimal String(number=w629) -> (decimal integer string=w627:string)  [unwired: 1 out]
              n229 = Concatenate Strings("BSA ", w627, " ") -> (w621:string)
              n230 = Concatenate Strings(w621, "Burst_Detector_Signal_to_Noise_Ratio" ("Pre Setup String")) -> (w624:string)
              n231 = Concatenate Strings(w621, "Level_Validation_Ratio" ("Pre Setup String")) -> (w622:string)
              n232 = call "Characters_to_string.vi"("Characters to write"=w623, "Label for characters"=w624) -> ("Output string"=w617:string)
              n233 = call "Characters_to_string.vi"("Characters to write"=w620, "Label for characters"=w622) -> ("Output string"=w618:string)
              n234 = Concatenate Strings(w617, w618) -> (w616:string)
            }
            frame #1 {
              n235 = Unbundle By Name(w646) -> ("Max Record length"=w638:u16, "Min Record length"=w640:u16, "Vel Comp"=w645:string, "Signal gain (dB)"=w644:i16, "High voltage"=w643:i16, "Max Velocity"=w642:dbl, "Min Velocity"=w641:dbl, "Optics Conversion Factor"=w635:dbl, "Multiply Velocity by -1"=w634:bool)  [unwired: 2 out]
              n236 = local read "Record Length"() -> (w637:dbl[])
              n237 = Index Array(array=w637, index=w638) -> (element=w636:dbl)
              n238 = Index Array(array=w637, index=w640) -> (element=w639:dbl)
              n239 = case shown="1" w633 {
                tunnel: w639 -> [w656 w666]
                tunnel: w645 -> [w655 w660]
                tunnel: w644 -> [w654 w661]
                tunnel: w643 -> [w653 w662]
                tunnel: w642 -> [w652 w663]
                tunnel: w641 -> [w651 w664]
                tunnel: w635 -> [w650 w665]
                tunnel: w636 -> [w649 w659]
                tunnel: w634 -> [w648 w658]
                tunnel: w632 -> [w647 w657]
                frame 0, Default {
                  n240 = global write "LDA_meas_global_1.vi" "Max Record length BSA1"(w649) -> ()
                  n241 = global write "LDA_meas_global_1.vi" "Optic Calib factor BSA1"(w650) -> ()
                  n242 = global write "LDA_meas_global_1.vi" "Additional BSA1 Setup"(w647) -> ()
                  n243 = global write "LDA_meas_global_1.vi" "Record length BSA1"(w656) -> ()
                  n244 = global write "LDA_meas_global_1.vi" "Multiply Velocity by -1"(w648) -> ()
                  n245 = global write "LDA_meas_global_1.vi" "Signal gain BSA1"(w654) -> ()
                  n246 = global write "LDA_meas_global_1.vi" "Vel Comp BSA1"(w655) -> ()
                  n247 = global write "LDA_meas_global_1.vi" "High Volt BSA1"(w653) -> ()
                  n248 = global write "LDA_meas_global_1.vi" "Max Vel BSA1"(w652) -> ()
                  n249 = global write "LDA_meas_global_1.vi" "Min Vel BSA1"(w651) -> ()
                }
                frame 1 {
                  n250 = global write "LDA_meas_global_2.vi" "Max Record length BSA2"(w659) -> ()
                  n251 = global write "LDA_meas_global_2.vi" "Optic Calib factor BSA2"(w665) -> ()
                  n252 = global write "LDA_meas_global_2.vi" "Additional BSA2 Setup"(w657) -> ()
                  n253 = global write "LDA_meas_global_2.vi" "Multiply Velocity by -1"(w658) -> ()
                  n254 = global write "LDA_meas_global_2.vi" "Record length BSA2"(w666) -> ()
                  n255 = global write "LDA_meas_global_2.vi" "Signal gain BSA2"(w661) -> ()
                  n256 = global write "LDA_meas_global_2.vi" "Vel Comp BSA2"(w660) -> ()
                  n257 = global write "LDA_meas_global_2.vi" "High Volt BSA2"(w662) -> ()
                  n258 = global write "LDA_meas_global_2.vi" "Max Vel BSA2"(w663) -> ()
                  n259 = global write "LDA_meas_global_2.vi" "Min Vel BSA2"(w664) -> ()
                }
              }
            }
          }
        }
      }
      frame "Close Panel" {
        n260 = Current VI's Path() -> (path=w669:path)
        n261 = call "Open_Close_Front_Panel.ph.vi"("Front Panel Window:Open"=FALSE, "VI path"=w669) -> ()  [unwired: 2 out]
      }
    }
    n262 = case shown="Error" w14 {
      tunnel: [w17 "Error"] -> w13
      tunnel: w12 -> [w17 _]
      frame No Error {
      }
      frame Error {
      }
    }
  }
